vi "SVT Unit Conversion (N Ch).vi"(0 "spectra":cluster{"x0":dbl, "dx":dbl, "magnitude":dbl[]}[](array[cluster]) {"magnitude" format="%.2p"; "dx" format="%.2p"; "x0" format="%.2p"}, 1 "desired scaling":T7 {"dB reference (0: no change)" format="%.2f"}, 2 "spectral density desired":T1(ring), 4 "spectrum info in":T2[](array[typedef]) {"x-axis units" items=["time"=0, "frequency"=1, "quefrency"=2, "revolutions"=3, "order"=4, "rpm"=11, "rad/s"=21, "index"=65535]; "weighting filter" items=["Linear", "A-weighting", "B-weighting", "C-weighting", "ITU-R 468-4", "Dolby", "CCITT", "C-message"]; "dB reference [EU]" format="%.2f"; "engineering units" items=["custom..."=0, "V"=1, "A"=21, "Pa"=2, "N"=20, "g"=3, "m/s^2"=4, "m/s"=5, "m"=6, "mm/s"=12, "mm"=13, "microns/s"=14, "microns"=15, "in/s^2"=7, "in/s"=8, "in"=9, "mils/s"=10, "mils"=11, "rad/s^2"=16, "rad/s"=17, "rad"=18, "strain"=19]; "spectral info"."window" items=["None "=0, "Hanning"=1, "Hamming"=2, "Blackman-Harris"=3, "Exact Blackman"=4, "Blackman"=5, "Flat Top"=6, "4 Term B-Harris "=7, "7 Term B-Harris"=8, "Low Sidelobe"=9, "Force - Exponential"=10, "Gaussian"=62]}, 5 "error in (no error)":errorcluster) -> (14 "converted spectra":cluster{"x0":dbl, "dx":dbl, "magnitude":dbl[]}[](array[cluster]) {"magnitude" format="%.2p"; "dx" format="%.2p"; "x0" format="%.2p"}, 15 "unit labels":string[](array[string]), 18 "spectrum info out":T2[](array[typedef]) {"x-axis units" items=["time"=0, "frequency"=1, "quefrency"=2, "revolutions"=3, "order"=4, "rpm"=11, "rad/s"=21, "index"=65535]; "weighting filter" items=["Linear", "A-weighting", "B-weighting", "C-weighting", "ITU-R 468-4", "Dolby", "CCITT", "C-message"]; "dB reference [EU]" format="%.2f"; "engineering units" items=["custom..."=0, "V"=1, "A"=21, "Pa"=2, "N"=20, "g"=3, "m/s^2"=4, "m/s"=5, "m"=6, "mm/s"=12, "mm"=13, "microns/s"=14, "microns"=15, "in/s^2"=7, "in/s"=8, "in"=9, "mils/s"=10, "mils"=11, "rad/s^2"=16, "rad/s"=17, "rad"=18, "strain"=19]; "spectral info"."window" items=["None "=0, "Hanning"=1, "Hamming"=2, "Blackman-Harris"=3, "Exact Blackman"=4, "Blackman"=5, "Flat Top"=6, "4 Term B-Harris "=7, "7 Term B-Harris"=8, "Low Sidelobe"=9, "Force - Exponential"=10, "Gaussian"=62]}, 19 "error out":errorcluster)   [LabVIEW 2017]
doc: "Converts between dB/linear, Magnitude/Magnitude^2, rms/peak/peak-peak, spectrum/spectral density, and dB ref1/dB ref2. You can use this polymorphic VI to convert a single spectrum, N spectra, a single complex spectrum, N complex spectra, a single channel of XY data, or N channels of XY data. The data type you wire to the <B>spectrum</B> input determines the polymorphic instance to use."
uses:
  <vilib>/addons/Sound and Vibration/compatibility/Controls/svl_Spectrum Info (enhanced).ctl
  <vilib>/addons/Sound and Vibration/compatibility/Controls/svl_Spectrum Type.ctl
  <vilib>/addons/Sound and Vibration/compatibility/Controls/svl_Engineering Units Text Ring.ctl
  <vilib>/addons/Sound and Vibration/compatibility/Controls/svl_Weighting Filter Text Ring.ctl
  <vilib>/addons/Sound and Vibration/compatibility/Controls/svl_Complimentary Spectrum Units.ctl
  <vilib>/addons/_NISVFA/_Shared subVIs/Common/svc_Spectrum Units.vi
  <vilib>/addons/_NISVFA/_Spectrum Processing/subVIs/svfa_Conversion Utility (spectrum info).vi
  <vilib>/addons/_NISVFA/_Spectrum Processing/subVIs/svfa_Peak to RMS to Peak2Peak.vi
  <vilib>/addons/_NISVFA/_Spectrum Processing/subVIs/svfa_Mag to Mag2.vi
  <vilib>/addons/_NISVFA/_Spectrum Processing/subVIs/svfa_Linear to dB.vi
  <vilib>/addons/_NISVFA/_Spectrum Processing/subVIs/svfa_dBrefA to dBrefB.vi
  <vilib>/addons/_NISVFA/_Spectrum Processing/subVIs/svfa_Spectrum to Spectral Density.vi
  <vilib>/addons/_NISVFA/_Shared subVIs/Common/svc_Get Weighting Enum and Labels.vi
  <vilib>/addons/_NISVFA/_Shared subVIs/Common/svc_Unit Label Lexical Class.vi
  <vilib>/addons/_NISVFA/_Shared subVIs/Common/svc_Engineering Units to Unit Label.vi
  <vilib>/addons/_NISVFA/_Shared subVIs/Common/svc_Format Value (DBL).vi
  <vilib>/addons/_NISVFA/_Shared subVIs/Common/svc_Window Parameters.vi
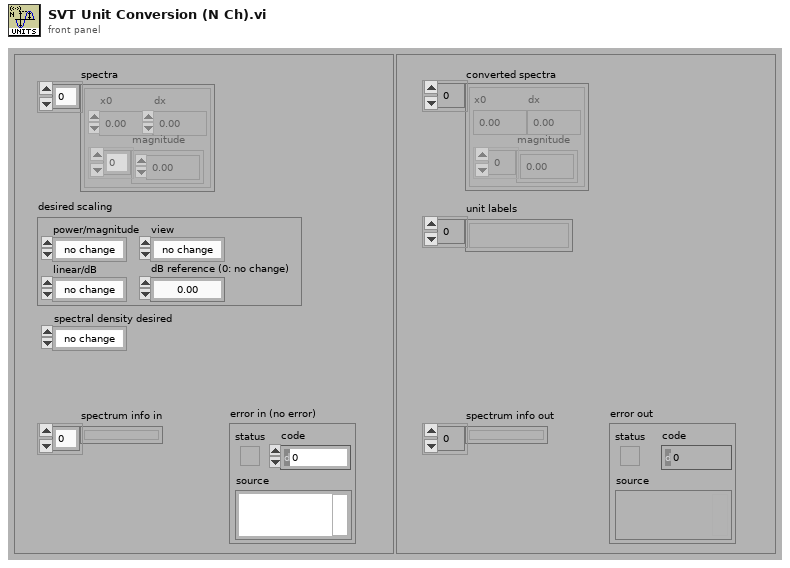
[diagram p1: front panel]
types:
  T1 = enum16{"no change", "spectrum", "spectral density"}
  T2 = typedef "svl_Spectrum Info (enhanced).ctl" = cluster{"channel name":string, "description":string, "x-axis units":u16, "spectral info":cluster{"spectrum type":T3, "linear/dB":enum16{"linear", "dB"}, "window":u16, "window size":i32, "FFT size":i32}, "engineering units":T4, "custom label":string, "dB reference [EU]":dbl, "peak units":enum16{"rms", "peak", "peak-peak"}, "weighting filter":T5, "spectral density?":bool, "unit label":string, "spectrum skewed?":bool, "complimentary spectrum units":T6}
  T3 = typedef "svl_Spectrum Type.ctl" = enum16{"FFT Spectrum [complex]", "Amplitude [Magnitude]", "Power [Magnitude^2]", "Cross Spectrum [complex]", "Frequency Response [Complex]"}
  T4 = typedef "svl_Engineering Units Text Ring.ctl" = u16
  T5 = typedef "svl_Weighting Filter Text Ring.ctl" = u16
  T6 = typedef "svl_Complimentary Spectrum Units.ctl" = enum16{"none", "radians", "degrees", "cycles", "imaginary"}
  T7 = cluster{"linear/dB":enum16{"no change", "linear", "dB"}, "dB reference (0: no change)":dbl, "power/magnitude":enum16{"no change", "power", "magnitude"}, "view":enum16{"no change", "rms", "peak", "peak-peak"}}
  T8 = typedef "svc_Spectrum Info.ctl" = cluster{"channel name":string, "description":string, "x-axis units":T9, "spectral info":cluster{"spectrum type":T10, "linear/dB":enum16{"linear", "dB"}, "window":u16, "window size":i32, "FFT size":i32}, "engineering units":T11, "custom label":string, "dB reference [EU]":dbl, "peak units":enum16{"rms", "peak", "peak-peak"}, "weighting filter":T12, "spectral density?":bool, "unit label":string, "spectrum skewed?":bool, "complimentary spectrum units":T13}
  T9 = typedef "svc_X-Axis Units.ctl" = u16
  T10 = typedef "svc_Spectrum Type.ctl" = enum16{"FFT Spectrum [complex]", "Amplitude [Magnitude]", "Power [Magnitude^2]", "Cross Spectrum [complex]", "Frequency Response [Complex]"}
  T11 = typedef "svc_Engineering Units Text Ring.ctl" = u16
  T12 = typedef "svc_Weighting Filter Text Ring.ctl" = u16
  T13 = typedef "svc_Complimentary Spectrum Units.ctl" = enum16{"none", "radians", "degrees", "cycles", "imaginary"}
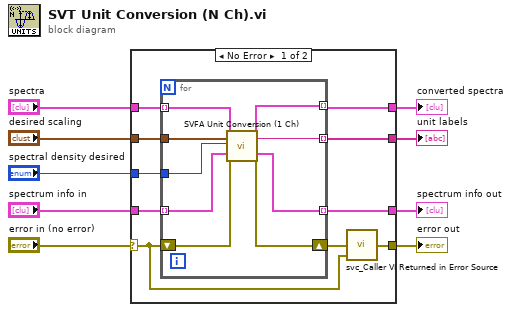
[diagram p0: block diagram]
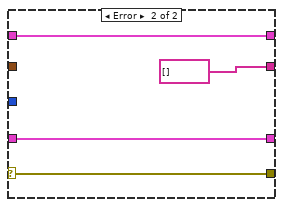
[diagram p2: hidden frame]
diagram:
  n1 = case shown="No Error" "error in (no error)" {
    selector: "error in (no error)" -> [w10 w32]
    tunnel: "spectrum info in" -> [w19 w31]
    tunnel: "spectra" -> [w18 w30]
    tunnel: "desired scaling" -> [w17 _]
    tunnel: [w12 w32] -> w6
    tunnel: [w15 w30] -> w5
    tunnel: [w14 w31] -> w4
    tunnel: [w13 string[] []] -> w3
    tunnel: "spectral density desired" -> [w11 _]
    frame No Error {
      n2 = for {
        tunnel: [w28] -> w15 mode=indexing
        shift-right: [w27] -> w16
        shift-left: w10 -> [w26]
        tunnel: w19 -> [w23] mode=indexing
        tunnel: w18 -> [w25] mode=indexing
        tunnel: w17 -> [w24]
        tunnel: [w22] -> w14 mode=indexing
        tunnel: [w21] -> w13 mode=indexing
        tunnel: w11 -> [w20]
        n3 = call <vilib>:"SVFA Unit Conversion (1 Ch).vi"("spectrum"=w25, "desired scaling"=w24, "spectral density desired"=w20, "spectrum info in"=w23, "error in (no error)"=w26) -> ("converted spectrum"=w28:cluster{"x0":dbl, "dx":dbl, "magnitude":dbl[]}, "unit label"=w21:string, "spectrum info out"=w22:T8, "error out"=w27:errorcluster)  [unwired: 11 in]
      }
      n4 = call <vilib>:"svc_Caller VI Returned in Error Source.vi"("warning input to caller"=w10, "error in (no error)"=w16) -> ("error out"=w12:errorcluster)  [unwired: 3 in]
    }
    frame Error {
    }
  }
  "error out" <- w6
  "spectrum info out" <- w4
  "converted spectra" <- w5
  "unit labels" <- w3
